vi "Watlow Global.vi"(7 "Write (F)":bool, 11 "Watlow Present":bool) -> (3 "Watlow Present OUT":bool)   [LabVIEW 2018]
panel:
  out "Watlow Present":bool
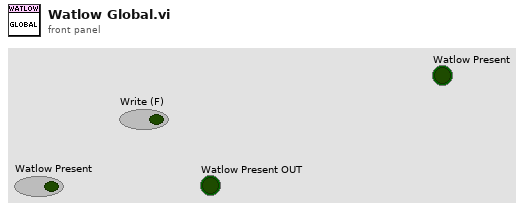
[diagram p1: front panel]
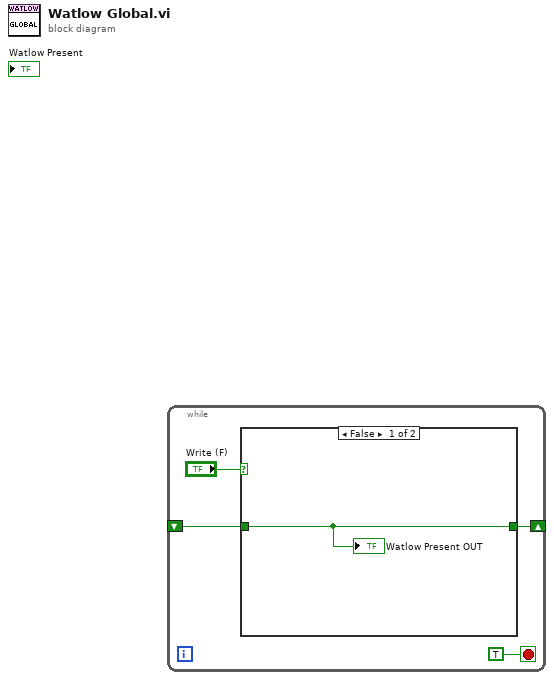
[diagram p0: block diagram]
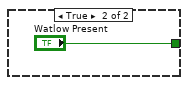
[diagram p2: hidden frame]
diagram:
  n1 = while {
    shift-right: [w2] -> _
    shift-left: _ -> [w1]
    stop <- TRUE stop-if-true
    n2 = case shown="False" "Write (F)" {
      tunnel: [w5 "Watlow Present"] -> w2
      tunnel: w1 -> [w5 _]
      frame False {
        "Watlow Present OUT" <- w5
      }
      frame True {
      }
    }
  }
